vi "Delete Buffer DVR.vi"(8 "error in (no error)":errorcluster, 11 "Waveform Receive in":refnum<class "Waveform Receive.lvclass">) -> (0 "error out":errorcluster)   [LabVIEW 2012, in "Waveform Data Logger Engine.lvlib" / "Waveform Receive.lvclass"]
uses:
  Waveform Receive.lvclass
  Waveform Receive.lvclass/Waveform Receive.ctl
  Buffer/Waveform Buffer/Waveform Buffer.lvclass
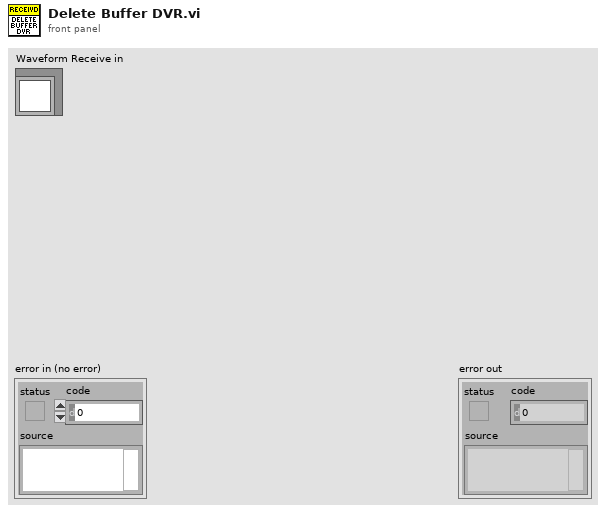
[diagram p1: front panel]
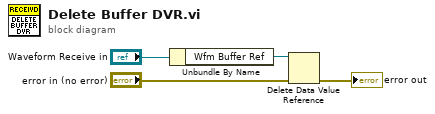
[diagram p0: block diagram]
diagram:
  n1 = Unbundle By Name("Waveform Receive in") -> ("Wfm Buffer Ref"=w2:refnum<data-value>)
  n2 = Delete Data Value Reference(data value reference=w2, error in="error in (no error)") -> (error out=→"error out":errorcluster)  [unwired: 1 out]
